vi "Read tag.vi"(8 "error in (no error)":errorcluster, 11 "Update CVT Data in":refnum<class "Update CVT Data.lvclass">) -> (0 "error out":errorcluster, 2 "tag":string, 3 "Update CVT Data out":refnum<class "Update CVT Data.lvclass">)   [LabVIEW 2014, in "Update CVT Data.lvclass"]
uses:
  Update CVT Data.lvclass
  Update CVT Data.lvclass/Update CVT Data.ctl
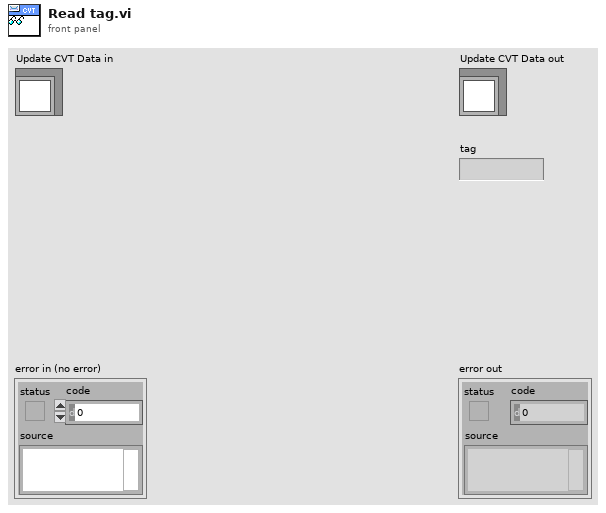
[diagram p1: front panel]
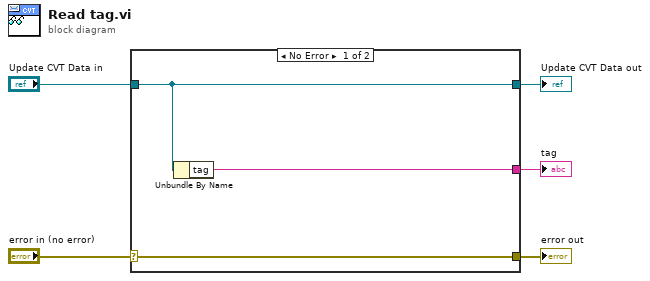
[diagram p0: block diagram]
diagram:
  n1 = case shown="No Error" "error in (no error)" {
    selector: "error in (no error)" -> [w8 w9]
    tunnel: [w8 w9] -> w4
    tunnel: [w7 w10] -> w2
    tunnel: "Update CVT Data in" -> [w7 w10]
    tunnel: [w6 _] -> w1
    frame No Error {
      n2 = Unbundle By Name(w7) -> ("tag"=w6:string)
    }
    frame Error {
    }
  }
  "error out" <- w4
  "Update CVT Data out" <- w2
  "tag" <- w1
